vi "Add ECAT Master.vi"(8 "error in (no error)":errorcluster, 11 "Parent Ref in":T1 format="%.0x") -> (0 "error out":errorcluster, 2 "Master Ref out":T1 format="%.0x", 3 "Parent Ref out":T1 format="%.0x")   [LabVIEW 2019, in "Scan Engine Custom Device.lvlib"]
uses:
  Scan Engine Custom Device.lvlib
  <vilib>/NI VeriStand/Custom Device API/Custom Device Item Ref.ctl
  Globals/Scan Engine GUIDs.vi
  Globals/Property Strings.vi
  <vilib>/NI VeriStand/Custom Device API/Custom Device API.lvlib
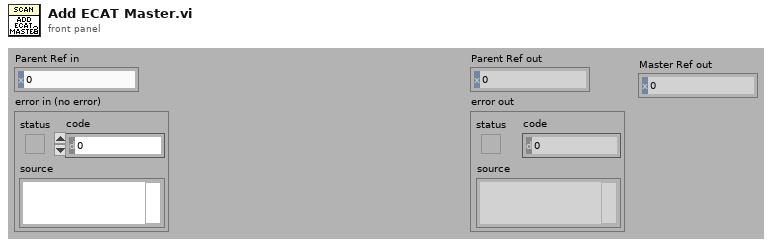
[diagram p1: front panel]
types:
  T1 = typedef "Custom Device API.lvlib/Custom Device Item Ref.ctl" = u64
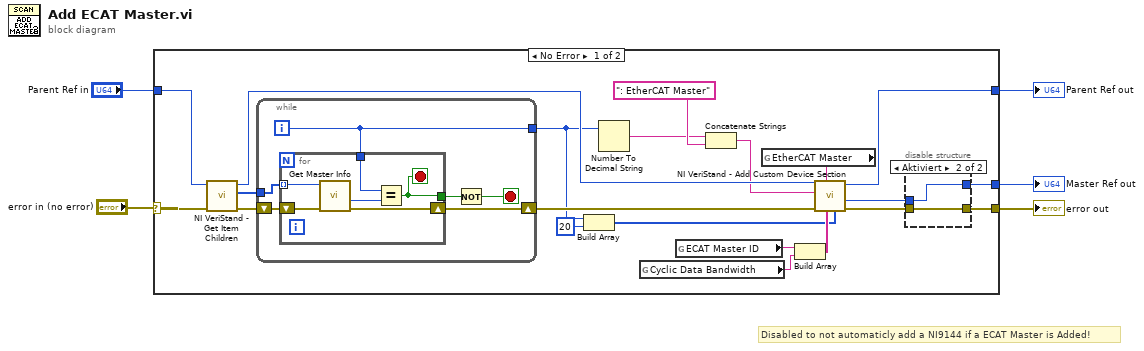
[diagram p0: block diagram]
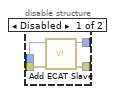
[diagram p2: hidden frame]
diagram:
  # "Disabled to not automaticly add a NI9144 if a ECAT Master is Added!"
  n1 = case shown="No Error" "error in (no error)" {
    selector: "error in (no error)" -> [w26 w46]
    tunnel: [w10 w46] -> w4
    tunnel: "Parent Ref in" -> [w25 w45]
    tunnel: [w12 w45] -> w2
    tunnel: [w8 _] -> w1
    frame No Error {
      n2 = call <vilib>:"NI VeriStand - Get Item Children.vi"("error in (no error)"=w26, "Item Ref in"=w25) -> ("error out"=w24:errorcluster, "Child Refs"=w23:T1[], "Item Ref out"=w20:T1)  [unwired: 6 in, 1 out]
      n3 = while {
        shift-right: [w34] -> w21
        shift-left: w24 -> [w38]
        tunnel: w23 -> [w37]
        tunnel: [w33] -> w16
        i -> [w33]
        stop <- w35 stop-if-true
        n4 = for {
          tunnel: w37 -> [w42] mode=indexing
          shift-right: [w40] -> w34
          shift-left: w38 -> [w41]
          tunnel: w33 -> [w44]
          tunnel: [w43] -> w36
          stop <- w43 stop-if-true
          n5 = call "Get Master Info.vi"("error in (no error)"=w41, "Item Ref in"=w42) -> ("error out"=w40:errorcluster, "Master #"=w39:u32)  [unwired: 6 in, 2 out]
          n6 = Equal?(x=w44, y=w39) -> (x = y?=w43:bool)
        }
        n7 = Not(x=w36) -> (.not. x?=w35:bool)
      }
      n8 = Build Array(w16, 20 ("element")) -> (w17:i32[])
      n9 = Number To Decimal String(number=w16) -> (decimal integer string=w14:string)  [unwired: 1 in]
      n10 = global read "Property Strings.vi" "Cyclic Data Bandwidth"() -> (w7:string)
      n11 = global read "Property Strings.vi" "ECAT Master ID"() -> (w19:string)
      n12 = Concatenate Strings(w14, ": EtherCAT Master" ("string")) -> (w13:string)
      n13 = global read "Scan Engine GUIDs.vi" "EtherCAT Master"() -> (w22:string)
      n14 = Build Array(w19, w7) -> (w18:string[])
      n15 = call <vilib>:"NI VeriStand - Add Custom Device Section.vi"("Property Values"=w17, "Property names"=w18, "GUID (Default Section)"=w22, "error in (no error)"=w21, "Section Name"=w13, "Parent Ref in"=w20) -> ("error out"=w11:errorcluster, "Section Ptr"=w9:T1, "Parent Ref out"=w12:T1)  [unwired: 2 in, 1 out]
      n16 = disable-structure shown="Aktiviert" {
        disable-tunnel: w11 -> [w30 w31]
        disable-tunnel: [w29 w31] -> w10
        disable-tunnel: w9 -> [w28 w32]
        disable-tunnel: [w27 w32] -> w8
        frame Disabled {
          n17 = call "Add ECAT Slave.vi"("error in (no error)"=w30, "ECAT Master Ref in"=w28) -> ("error out"=w29:errorcluster, "ECAT Master Ref out"=w27:T1)  [unwired: 8 in]
        }
        frame Enabled {
        }
      }
    }
    frame Error {
    }
  }
  "Parent Ref out" <- w2
  "error out" <- w4
  "Master Ref out" <- w1
